vi "am_read_subvi.vi"(7 "Aardvark Handle in":i32 min=0, 8 "error in (no error)":errorcluster, 9 "Address (0x50) in":u16=80 max=1023 format="%.0x", 10 "Num Bytes to Fetch (64)":u8=64 min=1, 11 "Memory ADD":u16=80 max=1023 format="%.0x") -> (0 "error out":errorcluster, 2 "Data byte":u8 format="%.0x", 3 "Dup Aardvark Handle":i32)   [LabVIEW 2014]
uses:
  aardvark.dll
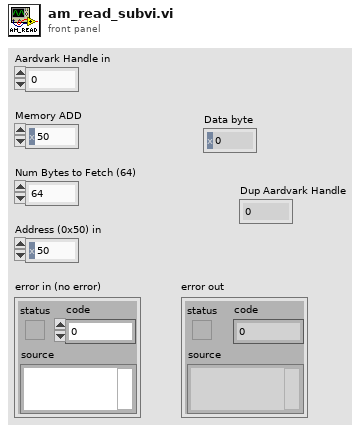
[diagram p1: front panel]
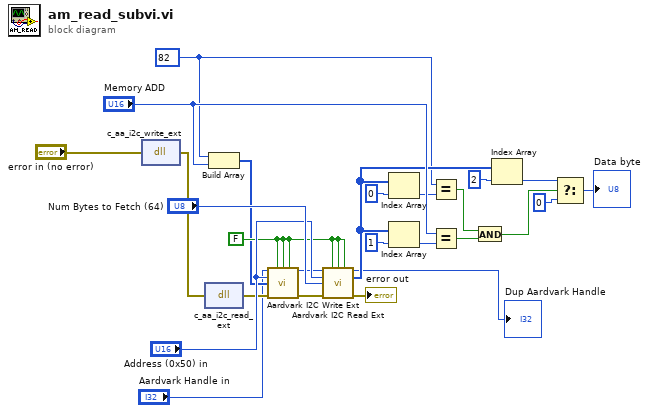
[diagram p0: block diagram]
diagram:
  w9 = FALSE
  w17 = u16 82
  n1 = dll-call lib="aardvark.dll" fn="c_aa_i2c_write_ext"(error in="error in (no error)") -> (error out=w5:errorcluster)  [unwired: 3 in, 1 out]
  n2 = dll-call lib="aardvark.dll" fn="c_aa_i2c_read_ext"(error in=w5) -> (error out=w8:errorcluster)  [unwired: 3 in, 1 out]
  n3 = Build Array(w17, "Memory ADD") -> (w7:u16[])
  n4 = call <instrlib>:"Aardvark I2C Write Ext.vi"("Aardvark Handle"="Aardvark Handle in", "10-bit Addressing? (False)"=w9, "Combined Format? (False)"=w9, "No Stop? (False)"=w9, "Address (0x50)"="Address (0x50) in", "Data to Write"=w7, "error in (no error)"=w8) -> ("dup Aardvark Handle"=w10:i32, "error out"=w13:errorcluster)  [unwired: 5 in, 2 out]
  n5 = call <instrlib>:"Aardvark I2C Read Ext.vi"("Aardvark Handle"=w10, "10-bit Addressing? (False)"=w9, "Combined Format? (False)"=w9, "No Stop? (False)"=w9, "Address (0x50)"="Address (0x50) in", "Num Bytes to Fetch (64)"="Num Bytes to Fetch (64)", "error in (no error)"=w13) -> ("dup Aardvark Handle"=→"Dup Aardvark Handle":i32, "Incoming Data"=w21:u8[], "error out"=→"error out":errorcluster)  [unwired: 5 in, 1 out]
  n6 = Index Array(array=w21, index=0) -> (element=w16:u8)
  n7 = Index Array(array=w21, index=1) -> (element=w19:u8)
  n8 = Equal?(x=w17, y=w16) -> (x = y?=w22:bool)
  n9 = Equal?(x="Memory ADD", y=w19) -> (x = y?=w23:bool)
  n10 = And(x=w22, y=w23) -> (x .and. y?=w25:bool)
  n11 = Index Array(array=w21, index=2) -> (element=w26:u8)
  n12 = Select(t=w26, s=w25, f=u8 0) -> (s? t:f=→"Data byte":u8)
